vi "Finish Move.vi"(8 "error in (no error)":errorcluster, 11 "SwipeScrollListbox in":refnum<class "SwipeScrollListbox.lvclass">) -> (0 "error out":errorcluster, 3 "SwipeScrollListbox out":refnum<class "SwipeScrollListbox.lvclass">)   [LabVIEW 2019, in "SwipeScrollListbox.lvclass"]
uses:
  SwipeScrollListbox.lvclass
  C:/Program Files (x86)/National Instruments/LabVIEW 2019/vi.lib/QSI/QControls/QControl Classes/ListBox/ListBox.lvclass
  SwipeScrollListbox.lvclass/SwipeScrollListbox.ctl
  <vilib>/Utility/inputDevices.llb/mouseAcquire.vi
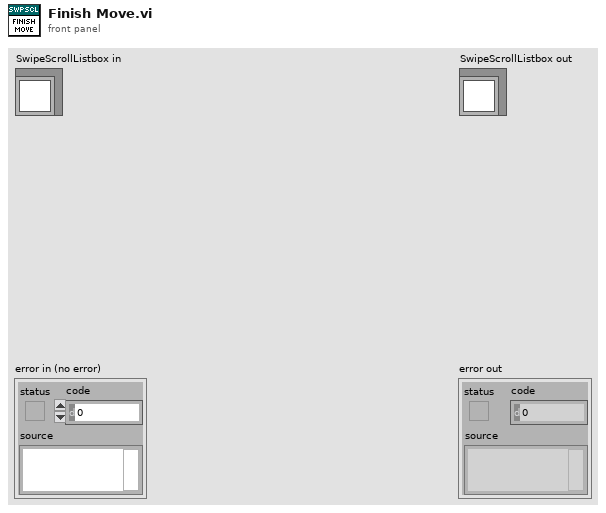
[diagram p1: front panel]
types:
  T1 = cluster{"Horizontal":i32, "Vertical":i32, "Scrolling":i32}
  T2 = typedef "SwipeScrollListbox.lvclass/State Data.ctl" = cluster{"Timeout":i32, "Time":timestamp, "Y":i32, "Slow Distance":i32, "Rate":dbl, "Row Selected":i32}
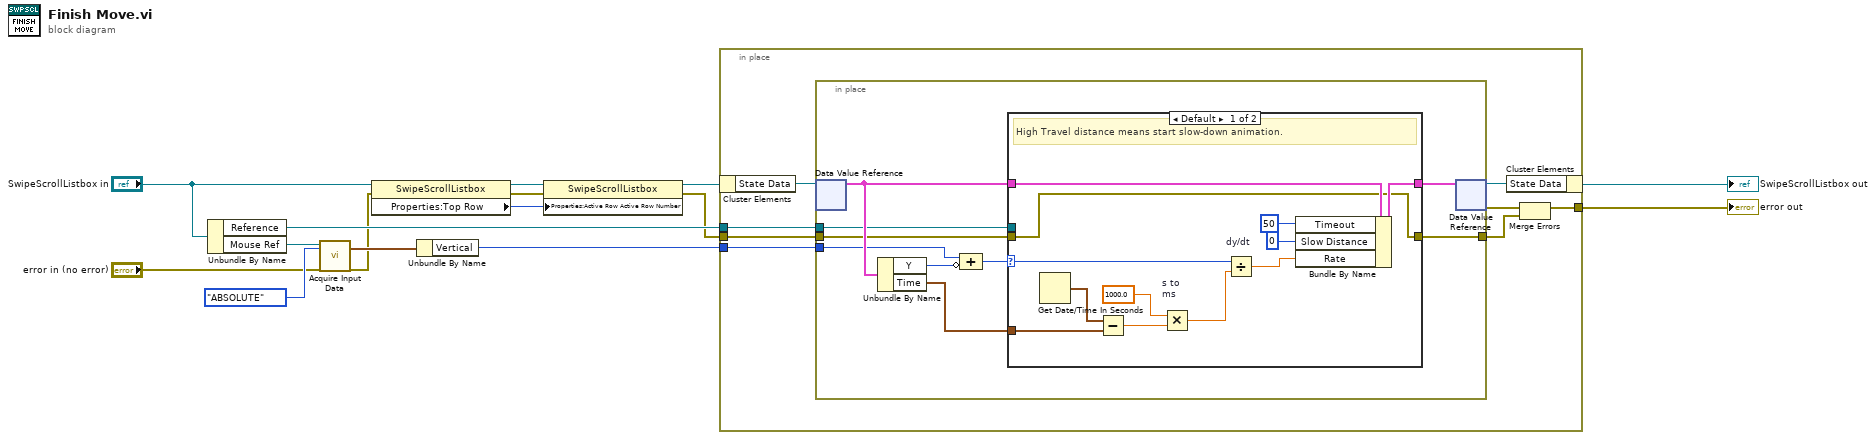
[diagram p0: block diagram]
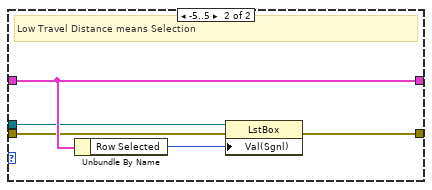
[diagram p2: hidden frame]
diagram:
  n1 = Unbundle By Name("SwipeScrollListbox in") -> ("Reference"=w3:refnum<vi>, "Mouse Ref"=w13:refnum<k1>)
  n2 = call-poly <vilib>:"Acquire Input Data.vi"("device ID"=w13, "key mode"=enum16{"RELATIVE", "ABSOLUTE"}."ABSOLUTE", "error in (no error)"="error in (no error)") -> ("axis info"=w14:T1, "error out"=w2:errorcluster)  [unwired: 13 in, 2 out]
  n3 = property class="SwipeScrollListbox"(reference="SwipeScrollListbox in", error in=w2) -> (reference out=w8:refnum<class "SwipeScrollListbox.lvclass">, error out=w7:errorcluster, "Properties:Top Row"=w6:i32)
  n4 = Unbundle By Name(w14) -> ("Vertical"=w10:i32)
  n5 = property class="SwipeScrollListbox"(reference=w8, error in=w7, "Properties:Active Row Active Row Number"=w6) -> (reference out=w4:refnum<class "SwipeScrollListbox.lvclass">, error out=w1:errorcluster)
  n6 = in-place {
    in-place-border: [w17] -> w9
    in-place-border: w10 -> [w20]
    in-place-border: w3 -> [w19]
    in-place-border: w1 -> [w18]
    n7 = in-place-cluster #1(w4) -> ("State Data"=w23:refnum<data-value>)
    n8 = in-place {
      in-place-border: w20 -> [w27]
      in-place-border: w19 -> [w26]
      in-place-border: w18 -> [w25]
      in-place-border: [w24] -> w16
      n9 = in-place-dvr #2(w23) -> (w31:T2)  [unwired: 1 out]
      n10 = Unbundle By Name(w31) -> ("Y"=w30:i32, "Time"=w28:timestamp)
      n11 = Compound Arithmetic op=ADD(w27, invert w30) -> (w29:i32)
      n12 = case shown="Default" w29 {
        selector: w29 -> [w41 _]
        tunnel: [w44 w49] -> w32
        tunnel: w31 -> [w42 w49]
        tunnel: w28 -> [w39 _]
        tunnel: w26 -> [_ w48]
        tunnel: w25 -> [w33 w46]
        tunnel: [w33 w45] -> w24
        frame Default {
          # "High Travel distance means start slow-down animation."
          n13 = Get Date/Time In Seconds() -> (seconds since 1Jan1904=w37:timestamp)
          n14 = Subtract(x=w37, y=w39) -> (x-y=w38:dbl)
          n15 = Multiply "s to\nms"(x=1000.0, y=w38) -> (x*y=w35:dbl)
          n16 = Divide "dy/dt"(x=w41, y=w35) -> (x/y=w40:dbl)
          n17 = Bundle By Name(cluster=w42, "Timeout"=50, "Slow Distance"=i16 0, "Rate"=w40) -> (w44:T2)
        }
        frame -5..5 {
          # "Low Travel Distance means Selection"
          n18 = Unbundle By Name(w49) -> ("Row Selected"=w47:i32)
          n19 = property class="LstBox"(reference=w48, error in=w46, "Val(Sgnl)"=w47) -> (error out=w45:errorcluster)  [unwired: 1 out]
        }
      }
      n20 = in-place-dvr #2(w32) -> (w22:refnum<data-value>, w21:errorcluster)
    }
    n21 = in-place-cluster #1("State Data"=w22) -> (→"SwipeScrollListbox out":refnum<class "SwipeScrollListbox.lvclass">)
    n22 = Merge Errors(w21, w16) -> (w17:errorcluster)
  }
  "error out" <- w9
